vi "Updater Copy PI Channel to New File.vi"(0 "Source tdms file in":refnum<k34>, 1 "Channel Name":string, 3 "Source Run ID":string, 5 "New tdms file in":refnum<k34>, 7 "New Run #":string, 11 "error out 4":errorcluster, 12 "error out":errorcluster) -> (4 "tdms file out 2":refnum<k34>, 8 "tdms file out 3":refnum<k34>, 14 "error out 3":errorcluster, 15 "error out 2":errorcluster)   [LabVIEW 2011]
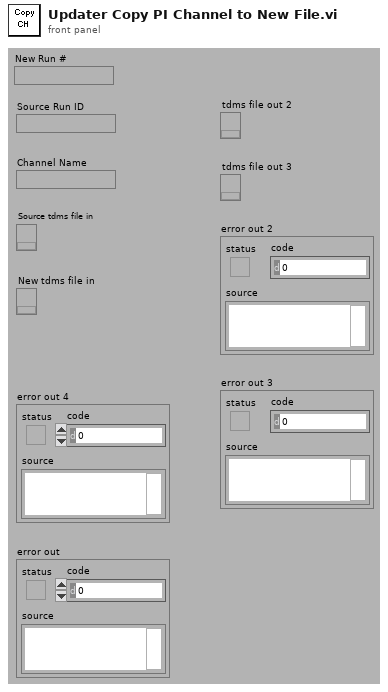
[diagram p1: front panel]
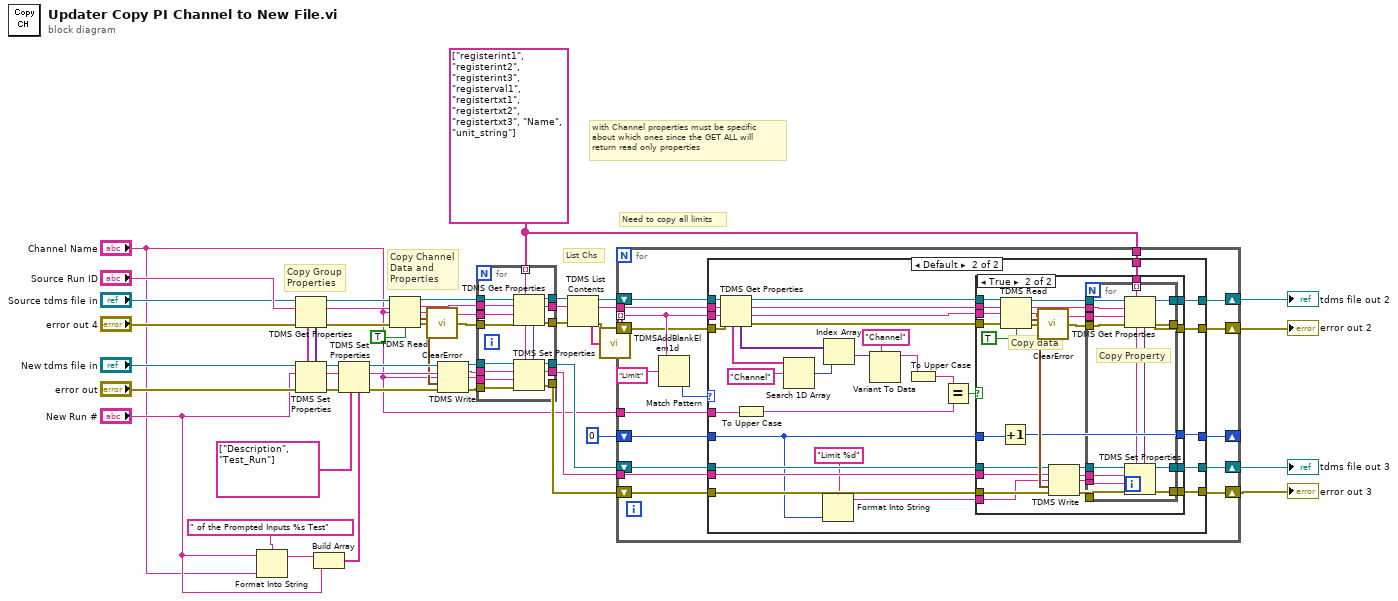
[diagram p0: block diagram]
diagram:
  w50 = string[] ["registerint1", "registerint2", "registerint3", "registerval1", "registertxt1", "registertxt2", "registertxt3", "Name", "unit_string"]
  # "Need to copy all limits"
  # "List Chs"
  # "with Channel properties must be specific\nabout which ones since the GET ALL will\nreturn read only properties"
  # "Copy Channel\nData and \nProperties"
  # "Copy Group\nProperties"
  n1 = Format Into String(format string=" of the Prompted Inputs %s Test" ("Field Internal ID"), initial string="New Run #", "Channel Name") -> (resulting string=w14:string)  [unwired: 1 in, 1 out]
  n2 = TDMS Get Properties(8:"error out 4", 10:"Source Run ID", 11:"Source tdms file in") -> (0:w12:errorcluster, 2:w27:string, 3:w11:refnum<k34>, 4:w10:variant[], 6:w9:string[])  [unwired: 4 out]
  n3 = TDMS Set Properties(5:w10, 7:w9, 8:"error out", 10:"New Run #", 11:"New tdms file in") -> (0:w21:errorcluster, 2:w16:string, 3:w15:refnum<k34>)  [unwired: 2 out]
  n4 = Build Array(w14, "New Run #") -> (w19:string[])
  n5 = TDMS Set Properties(5:w19, 7:string[] ["Description", "Test_Run"], 8:w21, 10:w16, 11:w15) -> (0:w22:errorcluster, 2:w17:string, 3:w20:refnum<k34>)  [unwired: 2 out]
  n6 = TDMS Read(0:w11, 5:w27, 7:"Channel Name", 11:w12, 13:TRUE ("return channels in file order? (F)")) -> (4:w25:refnum<k34>, 6:w28:string, 8:w29:string, 10:w8:waveform(dbl), 15:w2:errorcluster)  [unwired: 3 in, 1 out]
  n7 = call <vilib>:"ClearError.vi"("error in (no error)"=w2) -> ("error out"=w26:errorcluster)
  n8 = TDMS Write(0:w20, 5:w17, 7:"Channel Name", 9:w8, 11:w22) -> (4:w31:refnum<k34>, 6:w32:string, 8:w33:string, 15:w30:errorcluster)  [unwired: 1 in]
  n9 = for {
    tunnel: w25 -> [w66]
    tunnel: w26 -> [w65]
    tunnel: w28 -> [w64]
    tunnel: w29 -> [w63]
    tunnel: w30 -> [w62]
    tunnel: w31 -> [w61]
    tunnel: w32 -> [w59]
    tunnel: w33 -> [w58]
    tunnel: [w57] -> w34
    tunnel: [w56] -> w35
    tunnel: [w55] -> w36
    tunnel: [w54] -> w40
    tunnel: [w53] -> w41
    tunnel: [w52] -> w42
    tunnel: w50 -> [w51] mode=indexing
    n10 = TDMS Get Properties(7:w51, 8:w65, 9:w63, 10:w64, 11:w66) -> (0:w55:errorcluster, 2:w56:string, 3:w57:refnum<k34>, 4:w60:variant)  [unwired: 3 out]
    n11 = TDMS Set Properties(5:w60, 7:w51, 8:w62, 9:w58, 10:w59, 11:w61) -> (0:w52:errorcluster, 2:w53:string, 3:w54:refnum<k34>)  [unwired: 1 out]
  }
  n12 = TDMS List Contents(4:w36, 6:w35, 7:w34) -> (0:w46:errorcluster, 1:w3:string[], 2:w38:string, 3:w37:refnum<k34>)
  n13 = call <vilib>:"TDMSAddBlankElem1d.vi"("input string array"=w3) -> ("output string array with blank element at the beginning"=w23:string[])
  n14 = for {
    tunnel: w23 -> [w80] mode=indexing
    tunnel: w38 -> [w81]
    tunnel: "Channel Name" -> [w78]
    shift-right: [w73] -> _
    shift-left: 0 -> [w77]
    tunnel: w41 -> [w75]
    shift-right: [w67] -> w44
    shift-left: w42 -> [w74]
    shift-right: [w68] -> w43
    shift-left: w40 -> [w76]
    shift-right: [w70] -> w45
    shift-left: w37 -> [w82]
    shift-right: [w69] -> w47
    shift-left: w46 -> [w72]
    tunnel: w50 -> [w71]
    n15 = Match Pattern(string=w80, regular expression="Limit") -> (offset past match=w79:i32)  [unwired: 4 out]
    n16 = case shown="Default" w79 {
      tunnel: w82 -> [w87 w113]
      tunnel: w81 -> [_ w112]
      tunnel: w80 -> [_ w111]
      tunnel: w78 -> [_ w109]
      tunnel: w77 -> [w88 w90]
      tunnel: w76 -> [w85 w103]
      tunnel: w75 -> [_ w102]
      tunnel: [w84 w101] -> w67
      tunnel: w74 -> [w84 w100]
      tunnel: [w88 w89] -> w73
      tunnel: [w85 w99] -> w68
      tunnel: [w87 w98] -> w70
      tunnel: w72 -> [w86 w97]
      tunnel: [w86 w95] -> w69
      tunnel: w71 -> [_ w94]
      frame -1 {
        # "Not a limit channel"
      }
      frame Default {
        n17 = TDMS Get Properties(8:w97, 9:w111, 10:w112, 11:w113) -> (0:w96:errorcluster, 1:w104:string, 2:w105:string, 3:w106:refnum<k34>, 4:w117:variant[], 6:w119:string[])  [unwired: 2 out]
        n18 = To Upper Case(1:w109) -> (0:w107:string)
        n19 = Search 1D Array(1D array=w119, element="Channel") -> (index of element=w116:i32)  [unwired: 1 out]
        n20 = Format Into String(format string="Limit %d", w90) -> (resulting string=w92:string)  [unwired: 2 in, 1 out]
        n21 = Index Array(array=w117, index=w116) -> (element=w115:variant)
        n22 = Variant To Data(type="Channel", Variant=w115) -> (data=w110:string)  [unwired: 1 in, 1 out]
        n23 = To Upper Case(1:w110) -> (0:w108:string)
        n24 = Equal?(x=w108, y=w107) -> (x = y?=w91:bool)
        n25 = case shown="True" w91 {
          tunnel: w106 -> [w123 w141]
          tunnel: w105 -> [_ w140]
          tunnel: w104 -> [_ w139]
          tunnel: w103 -> [w121 w138]
          tunnel: w102 -> [_ w137]
          tunnel: [w120 w136] -> w101
          tunnel: w100 -> [w120 w135]
          tunnel: [w121 w134] -> w99
          tunnel: [w123 w133] -> w98
          tunnel: w96 -> [w122 w132]
          tunnel: [w122 w131] -> w95
          tunnel: w94 -> [_ w130]
          tunnel: w92 -> [_ w129]
          tunnel: w90 -> [w124 w128]
          tunnel: [w124 w127] -> w89
          frame False {
            # "This limit is not for the channel\nwe are processing."
          }
          frame True {
            # "Copy data"
            n26 = Increment(x=w128) -> (x+1=w127:i32)
            n27 = TDMS Read(0:w141, 5:w140, 7:w139, 11:w132, 13:TRUE ("return channels in file order? (F)")) -> (4:w143:refnum<k34>, 6:w145:string, 8:w146:string, 10:w142:waveform(dbl), 15:w126:errorcluster)  [unwired: 3 in, 1 out]
            n28 = call <vilib>:"ClearError.vi"("error in (no error)"=w126) -> ("error out"=w144:errorcluster)
            n29 = TDMS Write(0:w138, 5:w137, 7:w129, 9:w142, 11:w135) -> (4:w148:refnum<k34>, 6:w149:string, 8:w150:string, 15:w147:errorcluster)  [unwired: 1 in]
            n30 = for {
              tunnel: w150 -> [w164]
              tunnel: w149 -> [w163]
              tunnel: w148 -> [w161]
              tunnel: w147 -> [w160]
              tunnel: w146 -> [w159]
              tunnel: w145 -> [w158]
              tunnel: w144 -> [w157]
              tunnel: w143 -> [w156]
              tunnel: [w155] -> w136
              tunnel: [w154] -> w134
              tunnel: [w153] -> w133
              tunnel: [w152] -> w131
              tunnel: w130 -> [w151] mode=indexing
              # "Copy Property"
              n31 = TDMS Get Properties(7:w151, 8:w157, 9:w159, 10:w158, 11:w156) -> (0:w152:errorcluster, 3:w153:refnum<k34>, 4:w162:variant)  [unwired: 4 out]
              n32 = TDMS Set Properties(5:w162, 7:w151, 8:w160, 9:w164, 10:w163, 11:w161) -> (0:w155:errorcluster, 3:w154:refnum<k34>)  [unwired: 2 out]
            }
          }
        }
      }
    }
  }
  "error out 2" <- w47
  "tdms file out 2" <- w45
  "error out 3" <- w44
  "tdms file out 3" <- w43
